vi "_API_BINANCE_GET_USDT_FUTURES_ExchangeInfo.vi"(0 "BinanceAPI in":refnum<class "BinanceAPI_.lvclass">, 5 "exchangeInfo":cluster{"symbol (eg. BTCUSDT)":string}, 11 "error in (no error)":errorcluster) -> (4 "BinanceAPI out":refnum<class "BinanceAPI_.lvclass">, 6 "value":T1, 8 "Body":string, 14 "insideInfo":string, 15 "error out":errorcluster)   [LabVIEW 2022 SP3, in "BinanceAPI_.lvclass"]
doc: "https://binance-docs.github.io/apidocs/futures/en/#exchange-information"
uses:
  BinanceAPI_.lvclass
  BinanceAPI_.lvclass/BinanceAPI_.ctl
  <vilib>/regexp/Match Regular Expression.xnode
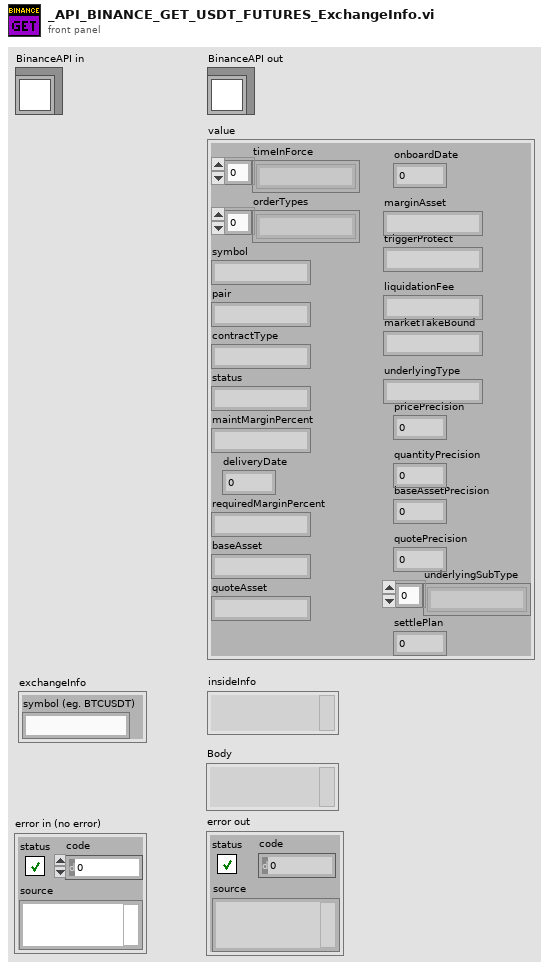
[diagram p1: front panel]
types:
  T1 = cluster{"timeInForce":string[], "orderTypes":string[], "symbol":string, "pair":string, "contractType":string, "status":string, "maintMarginPercent":string, "deliveryDate":dbl, "requiredMarginPercent":string, "baseAsset":string, "quoteAsset":string, "onboardDate":dbl, "marginAsset":string, "triggerProtect":string, "liquidationFee":string, "marketTakeBound":string, "underlyingType":string, "pricePrecision":dbl, "quantityPrecision":dbl, "baseAssetPrecision":dbl, "quotePrecision":dbl, "underlyingSubType":string[], "settlePlan":dbl}
  T2 = enum16{"SPOT", "USDT_FUTURES", "COIN_FUTURES", "VANILLA"}
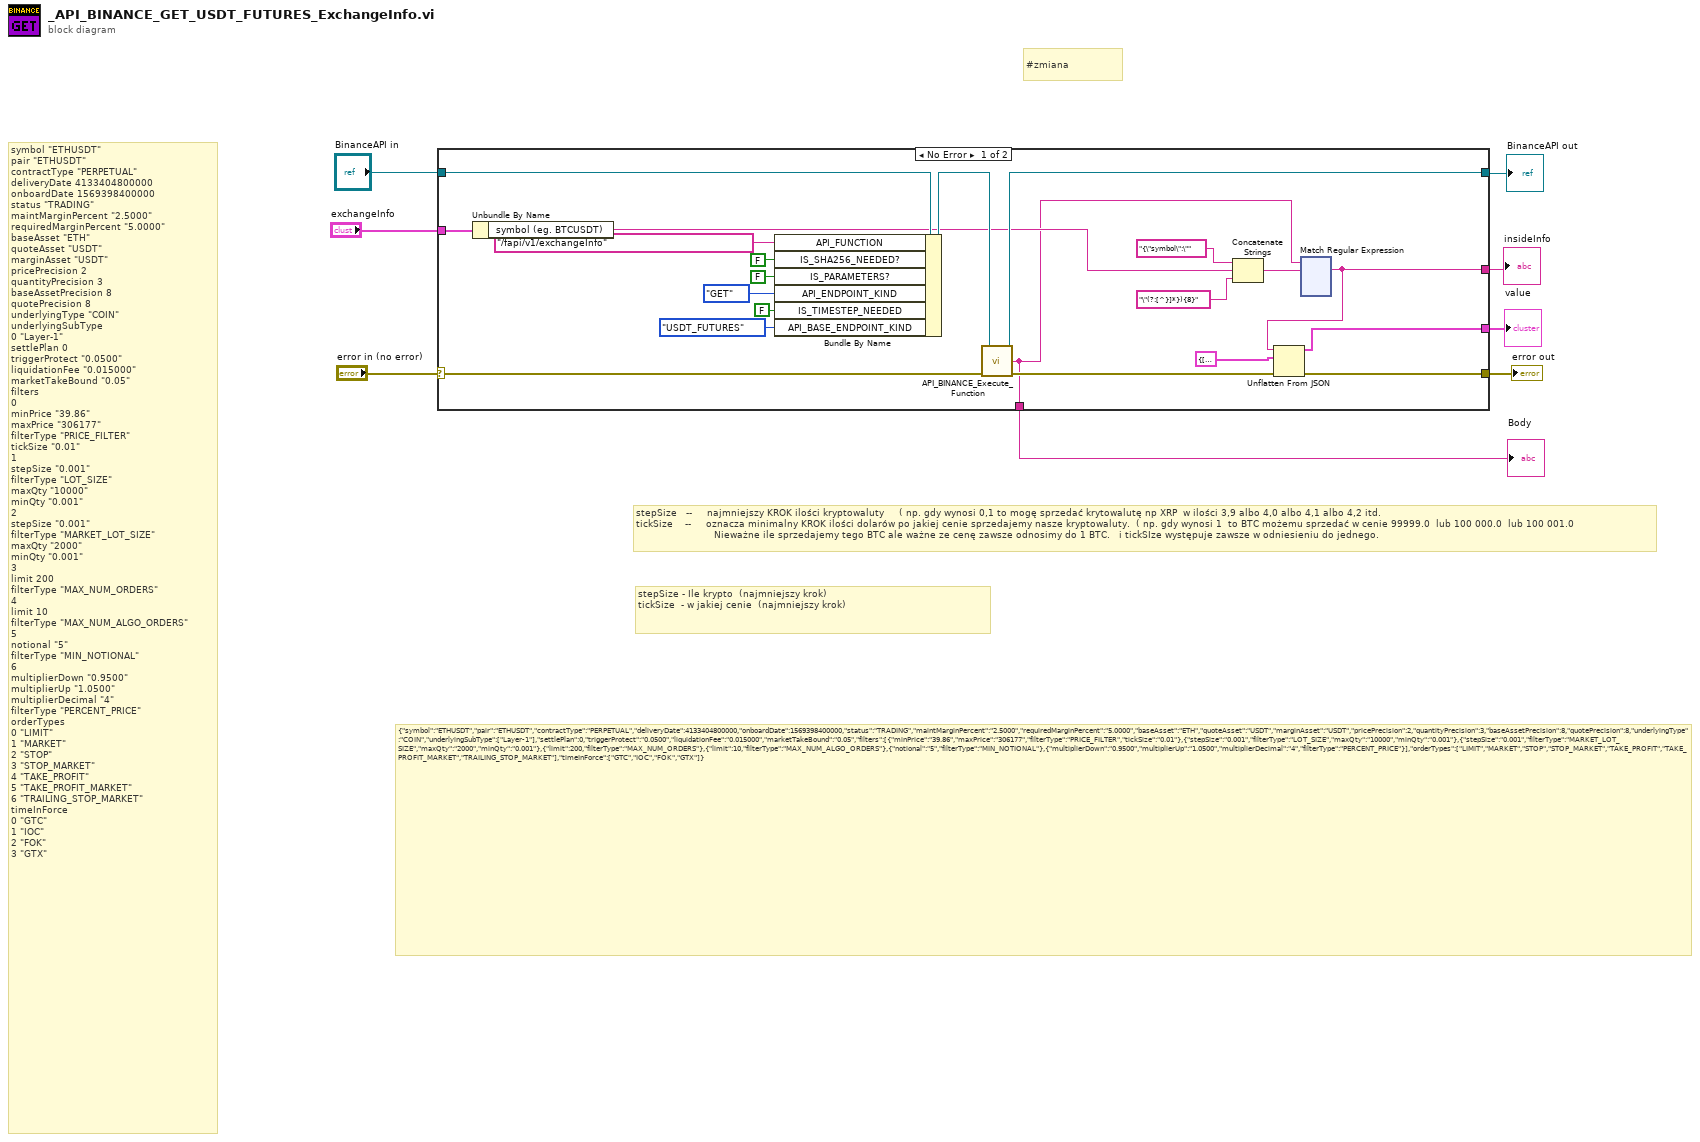
[diagram p0: block diagram]
diagram:
  # "symbol\t\"ETHUSDT\"\npair\t\"ETHUSDT\"\ncontractType\t\"PERPETUAL\"\ndeliveryDate\t4133404800000\nonboardDate\t1569398400000\nstatus\t\"TRADING\"\nmaintMarginPercent\t\"2.5000\"\nrequiredMarginPercent\t\"5.0000\"\nbaseAsset\t\"ETH\"\nquoteAsset\t\"USDT\"\nmarginAsset\t\"USDT\"\npricePrecision\t2\nquantityPrecision\t3\nbaseAssetPrecision\t8\nquotePrecision\t8\nunderlyingType\t\"COIN\"\nunderlyingSubType\t\n0\t\"Layer-1\"\nsettlePlan\t0\ntriggerProtect\t\"0.0500\"\nliquidationFee\t\"0.015000\"\nmarketTakeBound\t\"0.05\"\nfilters\t\n0\t\nminPrice\t\"39.86\"\nmaxPrice\t\"306177\"\nfilterType\t\"PRICE_FILTER\"\ntickSize\t\"0.01\"\n1\t\nstepSize\t\"0.001\"\nfilterType\t\"LOT_SIZE\"\nmaxQty\t\"10000\"\nminQty\t\"0.001\"\n2\t\nstepSize\t\"0.001\"\nfilterType\t\"MARKET_LOT_SIZE\"\nmaxQty\t\"2000\"\nminQty\t\"0.001\"\n3\t\nlimit\t200\nfilterType\t\"MAX_NUM_ORDERS\"\n4\t\nlimit\t10\nfilterType\t\"MAX_NUM_ALGO_ORDERS\"\n5\t\nnotional\t\"5\"\nfilterType\t\"MIN_NOTIONAL\"\n6\t\nmultiplierDown\t\"0.9500\"\nmultiplierUp\t\"1.0500\"\nmultiplierDecimal\t\"4\"\nfilterType\t\"PERCENT_PRICE\"\norderTypes\t\n0\t\"LIMIT\"\n1\t\"MARKET\"\n2\t\"STOP\"\n3\t\"STOP_MARKET\"\n4\t\"TAKE_PROFIT\"\n5\t\"TAKE_PROFIT_MARKET\"\n6\t\"TRAILING_STOP_MARKET\"\ntimeInForce\t\n0\t\"GTC\"\n1\t\"IOC\"\n2\t\"FOK\"\n3\t\"GTX\""
  # "{\"symbol\":\"ETHUSDT\",\"pair\":\"ETHUSDT\",\"contractType\":\"PERPETUAL\",\"deliveryDate\":4133404800000,\"onboardDate\":1569398400000,\"status\":\"TRADING\",\"maintMarginPercent\":\"2.5000\",\"requiredMarginPercent\":\"5.0000\",\"baseAsset\":\"ETH\",\"quoteAsset\":\"USDT\",\"marginAsset\":\"USDT\",\"pricePrecision\":2,\"quantityPrecision\":3,\"baseAssetPrecision\":8,\"quotePrecision\":8,\"underlyingType\":\"COIN\",\"underlyingSubType\":[\"Layer-1\"],\"settlePlan\":0,\"triggerProtect\":\"0.0500\",\"liquidationFee\":\"0.015000\",\"marketTakeBound\":\"0.05\",\"filters\":[{\"minPrice\":\"39.86\",\"maxPrice\":\"306177\",\"filterType\":\"PRICE_FILTER\",\"tickSize\":\"0.01\"},{\"stepSize\":\"0.001\",\"filterType\":\"LOT_SIZE\",\"maxQty\":\"10000\",\"minQty\":\"0.001\"},{\"stepSize\":\"0.001\",\"filterType\":\"MARKET_LOT_SIZE\",\"maxQty\":\"2000\",\"minQty\":\"0.001\"},{\"limit\":200,\"filterType\":\"MAX_NUM_ORDERS\"},{\"limit\":10,\"filterType\":\"MAX_NUM_ALGO_ORDERS\"},{\"notional\":\"5\",\"filterType\":\"MIN_NOTIONAL\"},{\"multiplierDown\":\"0.9500\",\"multiplierUp\":\"1.0500\",\"multiplierDecimal\":\"4\",\"filterType\":\"PERCENT_PRICE\"}],\"orderTypes\":[\"LIMIT\",\"MARKET\",\"STOP\",\"STOP_MARKET\",\"TAKE_PROFIT\",\"TAKE_PROFIT_MARKET\",\"TRAILING_STOP_MARKET\"],\"timeInForce\":[\"GTC\",\"IOC\",\"FOK\",\"GTX\"]}"
  # "#zmiana"
  # "stepSize - Ile krypto  (najmniejszy krok)\ntickSize  - w jakiej cenie  (najmniejszy krok)"
  # "stepSize   --     najmniejszy KROK ilości kryptowaluty     ( np. gdy wynosi 0,1 to mogę sprzedać krytowalutę np XRP  w ilości 3,9 albo 4,0 albo 4,1 albo 4,2 itd.\ntickSize    --     oznacza minimalny KROK ilości dolarów po jakiej cenie sprzedajemy nasze kryptowaluty.  ( np. gdy wynosi 1  to BTC możemu sprzedać w cenie 99999.0  lub 100 000.0  lub 100 001.0 \n                          Nieważne ile sprzedajemy tego BTC ale ważne ze cenę zawsze odnosimy do 1 BTC.   i tickSIze występuje zawsze w odniesieniu do jednego."
  n1 = case shown="No Error" "error in (no error)" {
    selector: "error in (no error)" -> [w21 w148]
    tunnel: [w12 w148] -> w6
    tunnel: [w22 w147] -> w1
    tunnel: "BinanceAPI in" -> [w29 w147]
    tunnel: "exchangeInfo" -> [w24 _]
    tunnel: [w9 _] -> w5
    tunnel: [w11 _] -> w4
    tunnel: [w10 _] -> w3
    frame No Error {
      n2 = Unbundle By Name(w24) -> ("symbol (eg. BTCUSDT)"=w17:string)
      n3 = Bundle By Name(cluster=w29, "API_FUNCTION"="/fapi/v1/exchangeInfo", "IS_SHA256_NEEDED?"=FALSE, "IS_PARAMETERS?"=FALSE, "API_ENDPOINT_KIND"=enum16{"POST", "DELETE", "GET", "PUT"}."GET", "IS_TIMESTEP_NEEDED"=FALSE, "API_BASE_ENDPOINT_KIND"=T2."USDT_FUTURES") -> (w23:refnum<class "BinanceAPI_.lvclass">)
      n4 = call "API_BINANCE_Execute_Function.vi"("BinanceAPI in"=w23, "error in (no error)"=w21) -> ("BinanceAPI out"=w22:refnum<class "BinanceAPI_.lvclass">, "Body"=w10:string, "error out"=w13:errorcluster)  [unwired: 9 in, 2 out]
      n5 = Concatenate Strings("{\"symbol\":\"" ("regular expression"), w17, "\"(?:[^}]*}){8}" ("regular expression")) -> (w15:string)
      n6 = xnode "Match Regular Expression"("input string"=w10, "regular expression"=w15) -> ("whole match"=w9:string)  [unwired: 4 in, 4 out]
      n7 = Unflatten From JSON(JSON string=w9, type and defaults=T1 {"timeInForce"=[], "orderTypes"=[], "symbol"="", "pair"="", "contractType"="", "status"="", "maintMarginPercent"="", "deliveryDate"=0.0, "requiredMarginPercent"="", "baseAsset"="", "quoteAsset"="", "onboardDate"=0.0, "marginAsset"="", "triggerProtect"="", "liquidationFee"="", "marketTakeBound"="", "underlyingType"="", "pricePrecision"=0.0, "quantityPrecision"=0.0, "baseAssetPrecision"=0.0, "quotePrecision"=0.0, "underlyingSubType"=[], "settlePlan"=0.0}, error in (no error)=w13) -> (value=w11:T1, error out=w12:errorcluster)  [unwired: 4 in]
    }
    frame Error {
    }
  }
  "error out" <- w6
  "insideInfo" <- w5
  "value" <- w4
  "Body" <- w3
  "BinanceAPI out" <- w1
